vi "Related To.vi"(11 "Relation in":refnum<class "Relation.lvclass">) -> (2 "Related To":string)   [LabVIEW 2020, in "Conditu2.lvlib" / "Columns.lvlib" / "Relation.lvclass"]
uses:
  Relation.lvclass
  Relation.lvclass/Relation.ctl
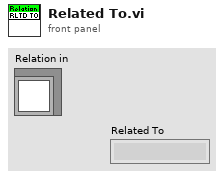
[diagram p1: front panel]
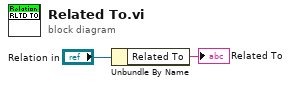
[diagram p0: block diagram]
diagram:
  n1 = Unbundle By Name("Relation in") -> ("Related To"=→"Related To":string)
